vi "ArrayOfTimeStamps.vi"() -> (0 "Array Of TimeStamps":timestamp[](array[timestamp]))   [LabVIEW 2013]
panel:
  in  "Time Stamp 3":timestamp=timestamp(3140113416 s since 1904-01-01)
  in  "Time Stamp 2":timestamp=timestamp(3137089404 s since 1904-01-01)
  in  "Time Stamp":timestamp=timestamp(3136484597 s since 1904-01-01)
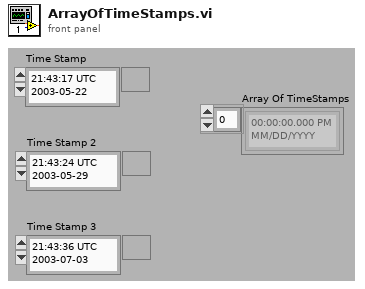
[diagram p1: front panel]
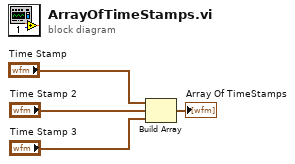
[diagram p0: block diagram]
diagram:
  n1 = Build Array("Time Stamp", "Time Stamp 2", "Time Stamp 3") -> (→"Array Of TimeStamps":timestamp[])
